vi "Do Apocalypse.vi"(11 "Start Notifier":refnum<notifier>) -> ()   [LabVIEW 2019]
doc: "This VI obtains a reference to every object on all open block diagrams, then destroys each by deleting it and replacing it with a fire graphic. The notifier controls when to begin deletion. All of the objects on a block diagram are deleted, a new block diagram is activated, and the process repeated."
uses:
  _Assets/Asset Enum.ctl
  c13ffa6b-2c19-41ec-ad78-a89946732768.vi
  <vilib>/numeric/Random Number (Range) U64.vi
  <vilib>/numeric/sub_Random U32.vi
  _Window/Window.lvlib
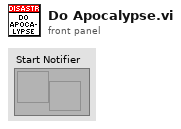
[diagram p1: front panel]
types:
  T1 = cluster{"BDWin.NativeWindow":u64, "vi reference":refnum<vi>}[]
  T2 = cluster{"vi reference":refnum<vi>, "Diagram":refnum<vi>, "shuffled array":refnum<vi>[]}
  T3 = typedef "Asset Enum.ctl" = enum16{"Fire 1", "Fire 2", "Rubble"}
  T4 = typedef "LVPositionTypeDef.ctl" = cluster{"Left":i32, "Top":i32}
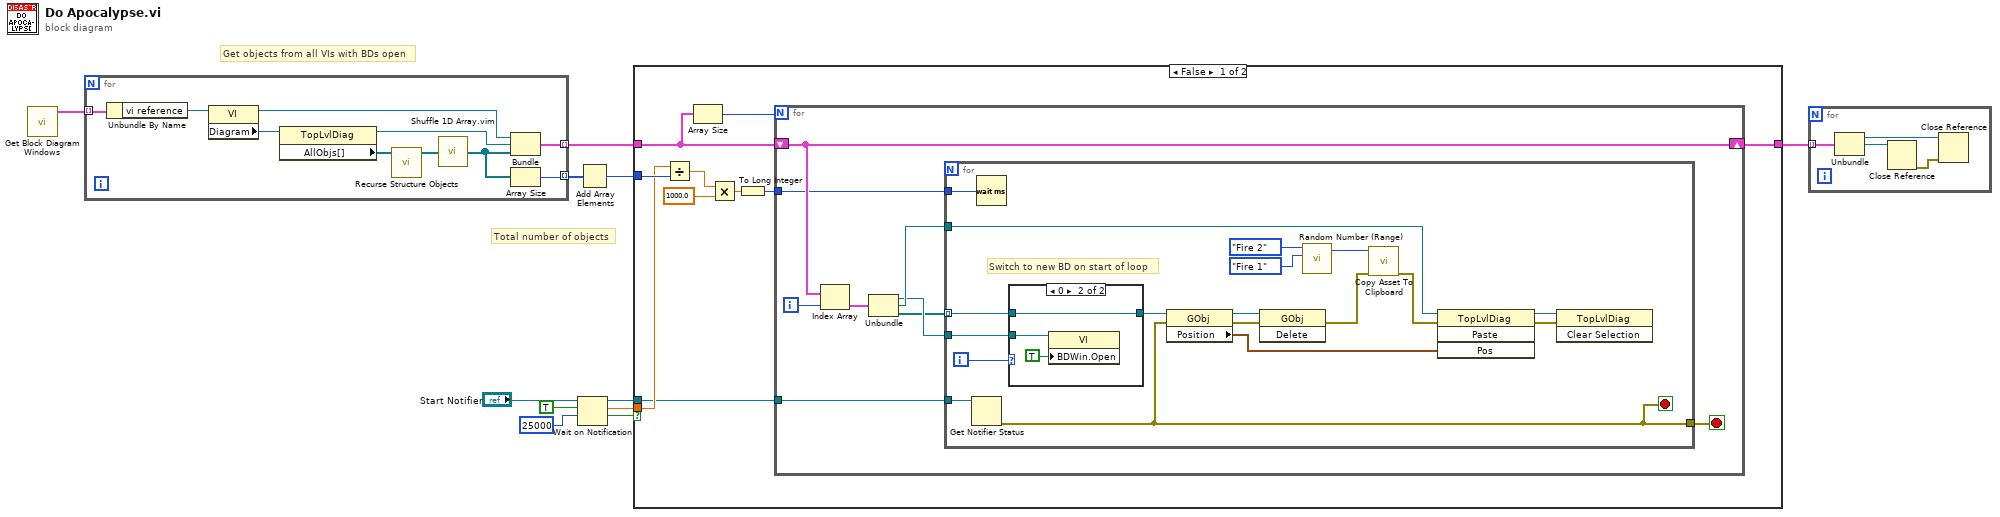
[diagram p0: block diagram]
diagram:
  # "Total number of objects"
  # "Get objects from all VIs with BDs open"
  n1 = call "Get Block Diagram Windows.vi"() -> ("VIs With Open BDs"=w11:T1)  [unwired: 11 in]
  n2 = for {
    tunnel: w11 -> [w19] mode=indexing
    tunnel: [w17] -> w9 mode=indexing
    tunnel: [w12] -> w7 mode=indexing
    n3 = Unbundle By Name(w19) -> ("vi reference"=w18:refnum<vi>)
    n4 = property class="VI"(reference=w18) -> (reference out=w15:refnum<vi>, "Diagram"=w20:refnum<vi>)  [unwired: 1 in, 1 out]
    n5 = property class="TopLvlDiag"(reference=w20) -> (reference out=w14:refnum<vi>, "AllObjs[]"=w21:refnum<vi>[])  [unwired: 1 in, 1 out]
    n6 = call "Recurse Structure Objects.vi"("Objects In"=w21) -> ("Objects Out"=w16:refnum<vi>[])  [unwired: 10 in]
    n7 = call "Shuffle 1D Array.vim"("array"=w16) -> ("shuffled array"=w13:refnum<vi>[])  [unwired: 4 in]
    n8 = Bundle("vi reference"=w15, "Diagram"=w14, "shuffled array"=w13) -> (w17:T2)  [unwired: 1 in]
    n9 = Array Size(array=w13) -> (size(s)=w12:i32)
  }
  n10 = Wait on Notification(notifier="Start Notifier", ignore previous (F)=TRUE, timeout in ms (-1)=25000) -> (notifier out=w3:refnum<notifier>, notification=w5:dbl, timed out?=w4:bool)  [unwired: 1 in, 1 out]
  n11 = Add Array Elements(numeric array=w7) -> (sum=w6:i32)
  n12 = case shown="False" w4 {
    tunnel: [w31 w63] -> w10
    tunnel: w9 -> [w30 w63]
    tunnel: w6 -> [w28 _]
    tunnel: w5 -> [w27 _]
    tunnel: w3 -> [w24 _]
    frame False {
      n13 = Divide(x=w27, y=w28) -> (x/y=w23:dbl)
      n14 = Array Size(array=w30) -> (size(s)=w29:i32)
      n15 = Multiply(x=w23, y=1000.0) -> (x*y=w25:dbl)
      n16 = To Long Integer(number=w25) -> (32bit integer=w22:i32)
      n17 = for {
        N: w29 -> [_]
        shift-right: [w35] -> w31
        shift-left: w30 -> [w35]
        tunnel: w22 -> [w34]
        tunnel: w24 -> [w33]
        i -> [w37]
        stop <- w32 stop-if-true
        n18 = Index Array(array=w35, index=w37) -> (element=w36:T2)
        n19 = Unbundle(w36) -> ("vi reference"=w39:refnum<vi>, "Diagram"=w40:refnum<vi>, "shuffled array"=w38:refnum<vi>[])
        n20 = for {
          tunnel: w38 -> [w49] mode=indexing
          tunnel: w39 -> [w47]
          tunnel: w34 -> [w45]
          tunnel: w33 -> [w44]
          tunnel: [w43] -> w32
          tunnel: w40 -> [w46]
          i -> [w48]
          stop <- w43 stop-if-true
          # "Switch to new BD on start of loop"
          n21 = Get Notifier Status(notifier=w44) -> (error out=w43:errorcluster)  [unwired: 1 in, 4 out]
          n22 = Wait (ms)(milliseconds to wait=w45) -> ()  [unwired: 1 out]
          n23 = case shown="0" w48 {
            tunnel: [w59 w62] -> w50
            tunnel: w49 -> [w59 w62]
            tunnel: w47 -> [_ w61]
            frame Default {
            }
            frame 0 {
              n24 = property class="VI"(reference=w61, "BDWin.Open"=TRUE ("Block Diagram Window:Open")) -> ()  [unwired: 1 in, 2 out]
            }
          }
          n25 = property class="GObj"(reference=w50, error in=w43) -> (reference out=w58:refnum<vi>, error out=w57:errorcluster, "Position"=w56:T4)
          n26 = invoke class="GObj" method="Delete"(reference=w58, error in=w57) -> (error out=w52:errorcluster)  [unwired: 1 in, 2 out]
          n27 = call-poly <vilib>:"Random Number (Range).vi"("lower bound (0)"=Asset_Enum."Fire 1" ("Asset"), "upper bound (100)"=Asset_Enum."Fire 2" ("Asset")) -> ("number"=w53:u64)  [unwired: 9 in]
          n28 = call "Copy Asset To Clipboard.vi"("error in (no error)"=w52, "Asset"=w53) -> ("error out"=w51:errorcluster)  [unwired: 9 in]
          n29 = invoke class="TopLvlDiag" method="Paste"(reference=w46, error in=w51, "Pos"=w56) -> (reference out=w42:refnum<vi>, error out=w41:errorcluster)  [unwired: 1 in, 2 out]
          n30 = invoke class="TopLvlDiag" method="Clear Selection"(reference=w42, error in=w41) -> ()  [unwired: 1 in, 3 out]
        }
      }
    }
    frame True {
    }
  }
  n31 = for {
    tunnel: w10 -> [w67] mode=indexing
    n32 = Unbundle(w67) -> ("vi reference"=w65:refnum<vi>, "Diagram"=w66:refnum<vi>)  [unwired: 1 out]
    n33 = Close Reference(reference=w66) -> (error out=w64:errorcluster)  [unwired: 1 in]
    n34 = Close Reference(reference=w65, error in (no error)=w64) -> ()  [unwired: 1 out]
  }
